vi "BotSpeak_Debug.vi"() -> ()   [LabVIEW 2012]
uses:
  <userlib>/BotSpeak/VIs/SubVIs/BotSpeak_Globals.vi
panel:
  in  "Tab Control":enum32{"TinySpeak", "Translated"}(tab)=enum."Translated"
  out "Current Buffer":string
  out "Translated Buffer":string
  in  "stop":bool
  in  "Abort?":bool
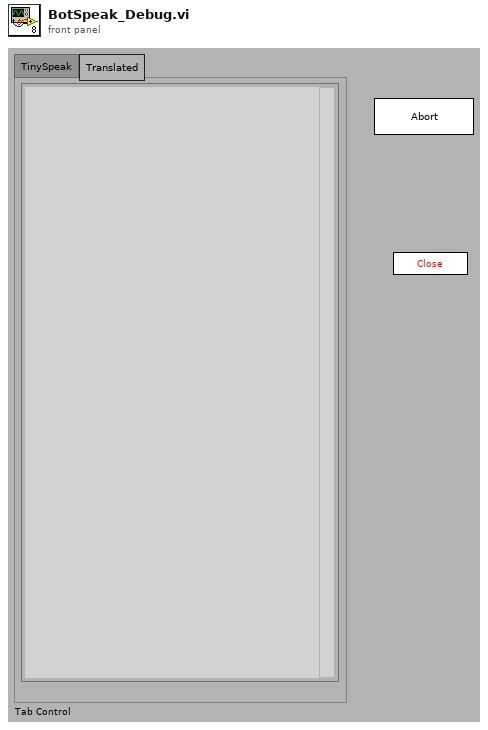
[diagram p1: front panel]
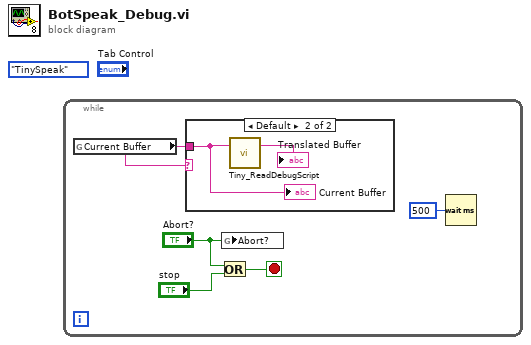
[diagram p0: block diagram]
diagram:
  (unwired) enum32{"TinySpeak", "Translated"}."TinySpeak" ("Tab Control")
  n1 = while {
    stop <- w2 stop-if-true
    n2 = global read "BotSpeak_Globals.vi" "Current Buffer"() -> (w1:string)
    n3 = case shown="Default" w1 {
      tunnel: w1 -> [_ w7]
      frame "" {
      }
      frame Default {
        n4 = call <userlib>:"Tiny_ReadDebugScript.vi"("read buffer"=w7) -> ("read buffer"=→"Translated Buffer":string)  [unwired: 2 in]
        "Current Buffer" <- w7
      }
    }
    n5 = Or(x="Abort?", y="stop") -> (x .or. y?=w2:bool)
    n6 = global write "BotSpeak_Globals.vi" "Abort?"("Abort?") -> ()
    n7 = Wait (ms)(milliseconds to wait=u32 500) -> ()  [unwired: 1 out]
  }
